vi "Startup.vi"() -> (0 "error out":errorcluster)   [LabVIEW 2020]
uses:
  <vilib>/Utility/EditLVProj/Edit LVProj.lvlib
  <resource>/objmgr/nisysapi.rc
panel:
  out "Tank":u8(slide) scale=0.0..6.0
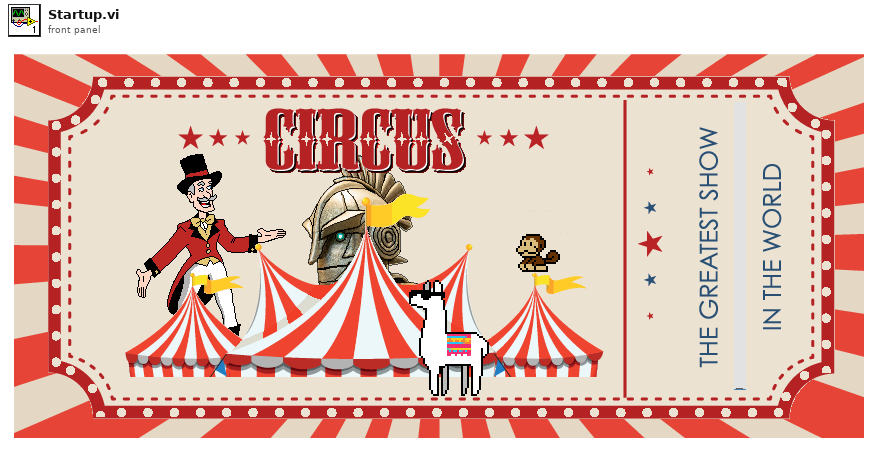
[diagram p1: front panel]
types:
  T1 = enum16{"open", "replace", "create", "open or create", "replace or create", "replace or create with confirmation"}
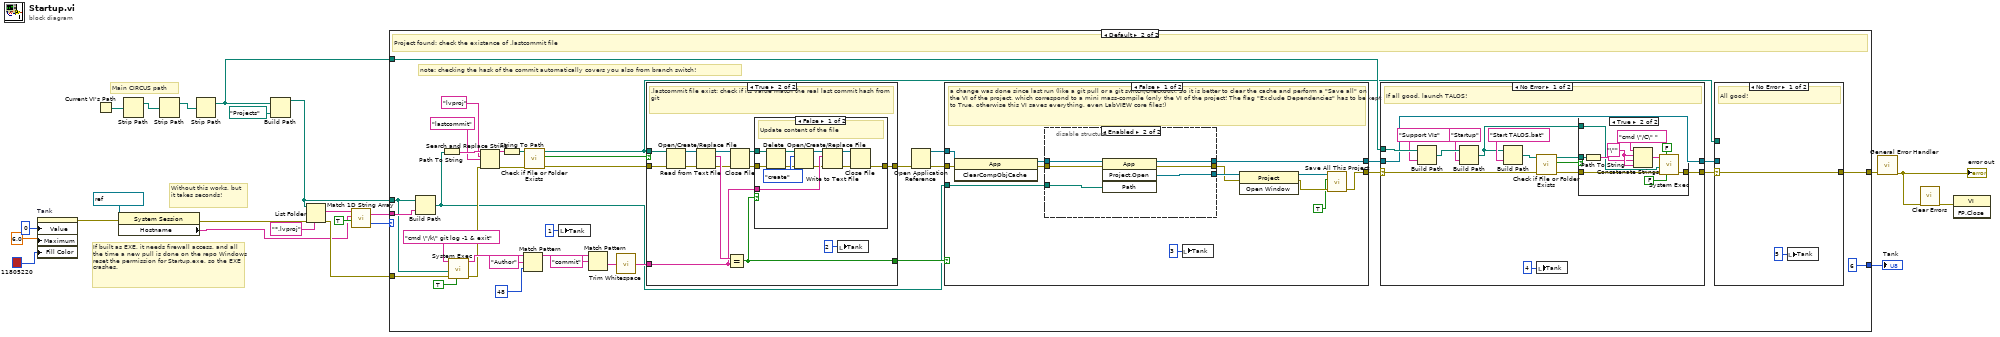
[diagram p0: block diagram]
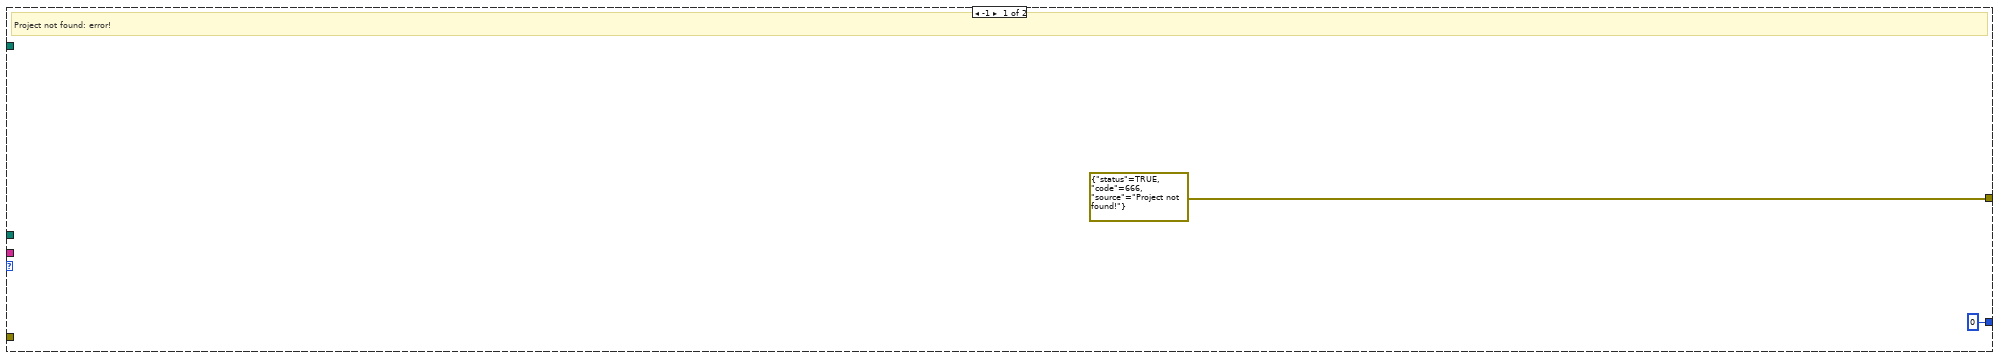
[diagram p2: hidden frame]
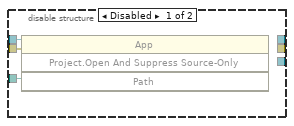
[diagram p3: hidden frame]
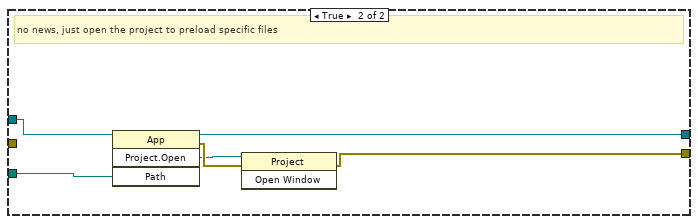
[diagram p4: hidden frame]
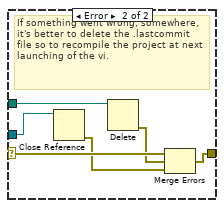
[diagram p5: hidden frame]
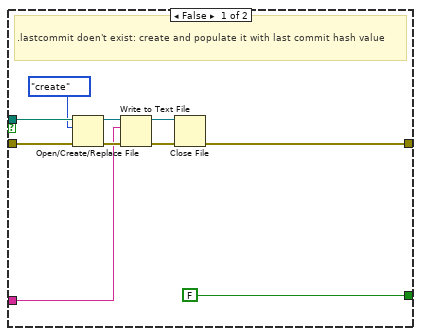
[diagram p6: hidden frame]
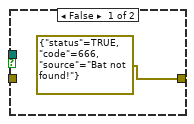
[diagram p8: hidden frame]
diagram:
  # "Without this works, but it takes seconds!"
  # "If built as EXE, it needs firewall access, and all the time a new pull is done on the repo Windows reset the permission for Startup.exe, so the EXE crashes."
  # "Main CIRCUS path"
  n1 = property on="Tank" class="Slide (strict)"("Value"=u8 0 ("Slide"), "Maximum"=6.0 ("Data Entry Limits:Maximum"), "Fill Color"=u32 11805220) -> (error out=w10:errorcluster)  [unwired: 2 in, 1 out]
  n2 = Current VI's Path() -> (path=w7:path)
  n3 = property class="System Session"(reference=refnum<k21> "localhost" ("System Session"), error in=w10) -> (error out=w14:errorcluster, "Hostname"=w13:string)  [unwired: 1 out]
  n4 = Strip Path(path=w7) -> (stripped path=w6:path)  [unwired: 1 out]
  n5 = Strip Path(path=w6) -> (stripped path=w5:path)  [unwired: 1 out]
  n6 = Strip Path(path=w5) -> (stripped path=w4:path)  [unwired: 1 out]
  n7 = Build Path(base path=w4, name or relative path=path "Projects") -> (appended path=w16:path)
  n8 = List Folder(path=w16, pattern="*.lvproj", error in=w14) -> (filenames=w22:string[], error out=w18:errorcluster)  [unwired: 1 in, 2 out]
  n9 = call <vilib>:"Match 1D String Array.vi"("Ignore Case? (false)"=TRUE, "Pattern"=w13, "Strings"=w22) -> ("index of element"=w19:i32, "Match"=w20:string)  [unwired: 1 in]
  n10 = case shown="Default" w19 {
    tunnel: w16 -> [_ w58]
    tunnel: w20 -> [_ w60]
    tunnel: w18 -> [_ w59]
    tunnel: [errorcluster {"status"=TRUE, "code"=666, "source"="Project not found!"} ("error IO") w36] -> w17
    tunnel: w4 -> [_ w37]
    tunnel: [u8 0 ("Slide") u8 6 ("Slide")] -> w2
    frame -1 {
      # "Project not found: error!"
    }
    frame Default {
      # "note: checking the hask of the commit automatically covers you also from branch switch!"
      # "Project found: check the existance of .lastcommit file"
      n11 = Build Path(base path=w58, name or relative path=w60) -> (appended path=w30:path)
      n12 = Path To String(path=w30) -> (string=w49:string)
      n13 = call <vilib>:"System Exec.vi"("run minimized? (F)"=TRUE, "error in (no error)"=w59, "working directory"=w58, "command line"="cmd \"/k\" git log -1 & exit") -> ("error out"=w40:errorcluster, "standard output"=w55:string)  [unwired: 4 in, 2 out]
      n14 = Search and Replace String(input string=w49, search string="lvproj" ("substring (\"\")"), replace string="lastcommit" ("replace string (\"\")"), error in=w40) -> (result string=w46:string, error out=w45:errorcluster)  [unwired: 4 in, 2 out]
      n15 = String To Path(string=w46) -> (path=w42:path)
      n16 = Match Pattern(string=w55, regular expression="Author", offset (0)=48) -> (before substring=w53:string)  [unwired: 3 out]
      n17 = call <vilib>:"Check if File or Folder Exists.vi"("error in (no error)"=w45, "path"=w42) -> ("error out"=w44:errorcluster, "file or folder exists?"=w41:bool, "dup path"=w35:path)  [unwired: 7 in]
      n18 = local write "Tank"(u8 1 ("Slide")) -> ()
      n19 = Match Pattern(string=w53, regular expression="commit") -> (after substring=w50:string)  [unwired: 1 in, 3 out]
      n20 = call <vilib>:"Trim Whitespace.vi"("string"=w50) -> ("trimmed string"=w43:string)  [unwired: 1 in]
      n21 = case shown="True" w41 {
        tunnel: w35 -> [w104 w119]
        tunnel: w43 -> [w99 w112]
        tunnel: w44 -> [w101 w118]
        tunnel: [FALSE w113] -> w32
        tunnel: [w98 w108] -> w39
        frame False {
          # ".lastcommit doen't exist: create and populate it with last commit hash value"
          n22 = Open/Create/Replace File(file path (use dialog)=w104, error in=w101, operation (0:open)=T1."create") -> (refnum out=w103:refnum<file>, error out=w105:errorcluster)  [unwired: 3 in, 1 out]
          n23 = Write to Text File(file (use dialog)=w103, text=w99, error in=w105) -> (refnum out=w102:refnum<file>, error out=w106:errorcluster)  [unwired: 1 in, 1 out]
          n24 = Close File(refnum=w102, error in=w106) -> (error out=w98:errorcluster)  [unwired: 1 out]
        }
        frame True {
          # ".lastcommit file exist: check if its value match the real last commit hash from git"
          n25 = Open/Create/Replace File(file path (use dialog)=w119, error in=w118) -> (refnum out=w117:refnum<file>, error out=w116:errorcluster)  [unwired: 4 in, 1 out]
          n26 = Read from Text File(file (use dialog)=w117, error in=w116) -> (refnum out=w114:refnum<file>, text=w115:string, error out=w111:errorcluster)  [unwired: 2 in, 1 out]
          n27 = Equal?(x=w115, y=w112) -> (x = y?=w113:bool)
          n28 = Close File(refnum=w114, error in=w111) -> (path=w109:path, error out=w110:errorcluster)
          n29 = case shown="False" w113 {
            tunnel: w110 -> [w126 w131]
            tunnel: w109 -> [w127 _]
            tunnel: [w120 w131] -> w108
            tunnel: w112 -> [w130 _]
            frame False {
              # "Update content of the file"
              n30 = Delete(path (use dialog)=w127, error in=w126) -> (deleted path=w124:path, error out=w123:errorcluster)  [unwired: 3 in, 1 out]
              n31 = Open/Create/Replace File(file path (use dialog)=w124, error in=w123, operation (0:open)=T1."create") -> (refnum out=w122:refnum<file>, error out=w121:errorcluster)  [unwired: 3 in, 1 out]
              n32 = Write to Text File(file (use dialog)=w122, text=w130, error in=w121) -> (refnum out=w128:refnum<file>, error out=w129:errorcluster)  [unwired: 1 in, 1 out]
              n33 = Close File(refnum=w128, error in=w129) -> (error out=w120:errorcluster)  [unwired: 1 out]
            }
            frame True {
              # "all good"
            }
          }
          n34 = local write "Tank"(u8 2 ("Slide")) -> ()
        }
      }
      n35 = Open Application Reference(8:w39) -> (0:w28:errorcluster, 3:w33:refnum<vi>)  [unwired: 3 in]
      n36 = case shown="False" w32 {
        tunnel: w30 -> [w73 w88]
        tunnel: [w66 w85] -> w29
        tunnel: w33 -> [w65 w84]
        tunnel: [w63 w83] -> w31
        tunnel: w28 -> [w62 _]
        frame False {
          # "a change was done since last run (like a git pull or a git switch/checkout). So it is better to clear the cache and perform a \"Save all\" on the VI of the project, which correspond to a mini mass-compile (only the VI of the project! The flag \"Exclude Dependencies\" has to be kept to True, otherwise this VI saves everything, even LabVIEW core files!)"
          n37 = invoke class="App" method="ClearCompObjCache"(reference=w65, error in=w62) -> (reference out=w64:refnum<vi>, error out=w72:errorcluster)  [unwired: 1 in, 1 out]
          n38 = disable-structure shown="Enabled" {
            disable-tunnel: w73 -> [w76 w82]
            disable-tunnel: w72 -> [w75 w81]
            disable-tunnel: [_ w80] -> w71
            disable-tunnel: [_ w79] -> w70
            disable-tunnel: w64 -> [w74 w78]
            disable-tunnel: [_ w77] -> w63
            frame Disabled {
              n39 = invoke class="App" method="Project.Open And Suppress Source-Only"(reference=w74, error in=w75, "Path"=w76) -> ()  [unwired: 1 in, 4 out]
            }
            frame Enabled {
              n40 = invoke class="App" method="Project.Open"(reference=w78, error in=w81, "Path"=w82) -> (reference out=w77:refnum<vi>, error out=w79:errorcluster, "Project:Open"=w80:refnum<vi>)  [unwired: 1 in, 1 out]
            }
          }
          n41 = local write "Tank"(u8 3 ("Slide")) -> ()
          n42 = invoke class="Project" method="Open Window"(reference=w71, error in=w70) -> (reference out=w69:refnum<vi>, error out=w68:errorcluster)  [unwired: 1 in, 1 out]
          n43 = call <vilib>:"Save All This Project.vi"("error in (no error)"=w68, "Exclude Dependencies? (F)"=TRUE, "Project in"=w69) -> ("error out"=w66:errorcluster)  [unwired: 7 in, 1 out]
        }
        frame True {
          # "no news, just open the project to preload specific files"
          n44 = invoke class="App" method="Project.Open"(reference=w84, "Path"=w88) -> (reference out=w83:refnum<vi>, error out=w87:errorcluster, "Project:Open"=w86:refnum<vi>)  [unwired: 2 in, 1 out]
          n45 = invoke class="Project" method="Open Window"(reference=w86, error in=w87) -> (error out=w85:errorcluster)  [unwired: 1 in, 2 out]
        }
      }
      n46 = case shown="No Error" w29 {
        selector: w29 -> [w144 w157]
        tunnel: [w143 w157] -> w38
        tunnel: w37 -> [w142 _]
        tunnel: w31 -> [w141 w156]
        tunnel: [w141 w156] -> w34
        frame No Error {
          # "If all good, launch TALOS!"
          n47 = Build Path(base path=w142, name or relative path="Support VIs") -> (appended path=w137:path)
          n48 = Build Path(base path=w137, name or relative path="Startup") -> (appended path=w135:path)
          n49 = Build Path(base path=w135, name or relative path="Start TALOS.bat") -> (appended path=w134:path)
          n50 = local write "Tank"(u8 4 ("Slide")) -> ()
          n51 = call <vilib>:"Check if File or Folder Exists.vi"("error in (no error)"=w144, "path"=w134) -> ("error out"=w133:errorcluster, "file or folder exists?"=w132:bool)  [unwired: 7 in, 1 out]
          n52 = case shown="True" w132 {
            tunnel: w134 -> [_ w155]
            tunnel: w133 -> [_ w154]
            tunnel: [errorcluster {"status"=TRUE, "code"=666, "source"="Bat not found!"} ("error out") w153] -> w143
            tunnel: w135 -> [_ w147]
            frame False {
            }
            frame True {
              w152 = "\"" ("string")
              n53 = Path To String(path=w155) -> (string=w150:string)
              n54 = Concatenate Strings("cmd \"/C\" " ("string"), w152, w150, w152) -> (w149:string)
              n55 = call <vilib>:"System Exec.vi"("run minimized? (F)"=FALSE, "wait until completion? (T)"=FALSE, "error in (no error)"=w154, "working directory"=w147, "command line"=w149) -> ("error out"=w153:errorcluster)  [unwired: 3 in, 3 out]
            }
          }
        }
        frame Error {
          # "something went wrong!"
        }
      }
      n56 = case shown="No Error" w38 {
        selector: w38 -> [w90 w95]
        tunnel: [w90 w93] -> w36
        tunnel: w35 -> [_ w96]
        tunnel: w34 -> [_ w94]
        frame No Error {
          # "All good!"
          n57 = local write "Tank"(u8 5 ("Slide")) -> ()
        }
        frame Error {
          # "If something went wrong, somewhere, it's better to delete the .lastcommit file so to recompile the project at next launching of the vi."
          n58 = Close Reference(reference=w94) -> (error out=w91:errorcluster)  [unwired: 1 in]
          n59 = Delete(path (use dialog)=w96) -> (error out=w92:errorcluster)  [unwired: 4 in, 2 out]
          n60 = Merge Errors(w95, w92, w91) -> (w93:errorcluster)
        }
      }
    }
  }
  "Tank" <- w2
  n61 = call <vilib>:"General Error Handler.vi"("error in (no error)"=w17) -> ("error out"=w12:errorcluster)  [unwired: 10 in, 4 out]
  "error out" <- w12
  n62 = call <vilib>:"Clear Errors.vi"("error in (no error)"=w12) -> ("error out"=w11:errorcluster)  [unwired: 5 in, 1 out]
  n63 = invoke class="VI" method="FP.Close"(error in=w11) -> ()  [unwired: 2 in, 3 out]
